vi "ObtainBroadcastForRegistration.vi"(8 "error in (no error)":errorcluster) -> (0 "error out":errorcluster, 2 "clDigitizerBdcstEvents":T1)   [LabVIEW 2014, in "DigitizerModule.lvlib"]
uses:
  DigitizerModule.lvlib
  Protected/Broadcasts/clBroadcastEvents.ctl
  Protected/clEventType.ctl
panel:
  # "Rename this for each module type"
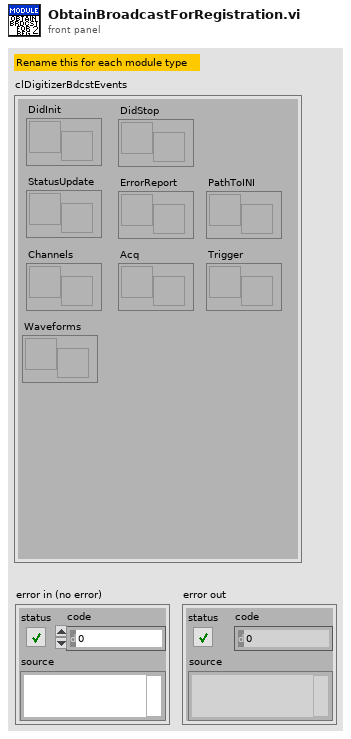
[diagram p1: front panel]
types:
  T1 = typedef "DigitizerModule.lvlib/clBroadcastEvents.ctl" = cluster{"DidInit":refnum<user-event>, "StatusUpdate":refnum<user-event>, "ErrorReport":refnum<user-event>, "DidStop":refnum<user-event>, "PathToINI":refnum<user-event>, "Channels":refnum<user-event>, "Acq":refnum<user-event>, "Trigger":refnum<user-event>, "Waveforms":refnum<user-event>}
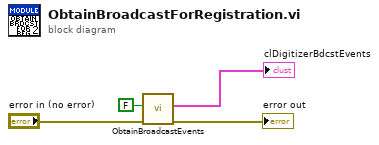
[diagram p0: block diagram]
diagram:
  n1 = call "ObtainBroadcastEvents.vi"("error in (no error)"="error in (no error)", "CreateNew? (F)"=FALSE) -> ("error out"=→"error out":errorcluster, "clDigitizerBdcstEvents"=→"clDigitizerBdcstEvents":T1)  [unwired: 8 in]
